vi "sv_Check for Even-Angle Signal.vi"(0 "data to process":waveform(dbl)[](array[waveform]), 11 "error in (no error)":errorcluster) -> (4 "data to process out":waveform(dbl)[](array[waveform]), 6 "even-angle signals":cluster{"r0":dbl, "dr":dbl, "Y":dbl[]}[](array[cluster]), 8 "even-angle channel info":T1[](array[typedef]) {"channel info"."pregain" format="%.2f"; "channel info"."weighting filter" items=["Linear", "A-weighting", "B-weighting", "C-weighting", "ITU-R 468-4", "Dolby", "CCITT", "C-message", "Wb", "Wc", "Wd", "We", "Wf", "Wh", "Wj", "Wk", "Wm", "AES17 20 kHz lowpass", "AES17 40 kHz lowpass", "AES17 20 kHz highpass", "AES17 40 kHz highpass"]; "channel info"."dB reference" format="%^.1e"; "channel info"."engineering units" items=["custom..."=0, "V"=1, "A"=21, "C"=30, "pC"=31, "s"=32, "-"=29, "Pa"=2, "N"=20, "g"=3, "m/s^2"=4, "m/s"=5, "m"=6, "mm/s"=12, "mm"=13, "micron/s"=14, "micron"=15, "in/s^2"=7, "in/s"=8, "in"=9, "mil/s"=10, "mil"=11, "rad/s^2"=16, "rad/s"=17, "rad"=18, "deg/s^2"=26, "deg/s"=27, "deg"=28, "RPM"=22, "cycle/s^2"=23, "Hz"=24, "cycle"=25, "strain"=19]; "channel info"."sensor sensitivity" format="%#_5f"}, 10 "even-angle position info":T5, 14 "found":bool, 15 "error out":errorcluster)   [LabVIEW 2017, in "SoundVib_ContSweptSine.lvlib"]
uses:
  <vilib>/addons/Sound and Vibration/svt_Continuous Swept Sine/SoundVib_ContSweptSine.lvlib
  <vilib>/addons/_NISVFA/_Shared subVIs/Controls/svc_Resampled Channel Info.ctl
  <vilib>/addons/_NISVFA/_Shared subVIs/Controls/svc_Channel Info.ctl
  <vilib>/addons/_NISVFA/_Shared subVIs/Controls/svc_Engineering Units Text Ring.ctl
  <vilib>/addons/_NISVFA/_Shared subVIs/Controls/svc_Weighting Filter Text Ring.ctl
  <vilib>/addons/Sound and Vibration/Order Analysis/Misc/OAT Position Info.ctl
  <vilib>/addons/Sound and Vibration/svt_Continuous Swept Sine/subVIs/sv_Continuous Swept-Sine Tags.ctl
  <vilib>/addons/Sound and Vibration/svt_Continuous Swept Sine/subVIs/sv_Continuous Swept-Sine Errors.ctl
panel:
  in  "even-angle position info":T5
  in  "even-angle channel info":T1[](array[typedef]) {"channel info"."pregain" format="%.2f"; "channel info"."weighting filter" items=["Linear", "A-weighting", "B-weighting", "C-weighting", "ITU-R 468-4", "Dolby", "CCITT", "C-message", "Wb", "Wc", "Wd", "We", "Wf", "Wh", "Wj", "Wk", "Wm", "AES17 20 kHz lowpass", "AES17 40 kHz lowpass", "AES17 20 kHz highpass", "AES17 40 kHz highpass"]; "channel info"."dB reference" format="%^.1e"; "channel info"."engineering units" items=["custom..."=0, "V"=1, "A"=21, "C"=30, "pC"=31, "s"=32, "-"=29, "Pa"=2, "N"=20, "g"=3, "m/s^2"=4, "m/s"=5, "m"=6, "mm/s"=12, "mm"=13, "micron/s"=14, "micron"=15, "in/s^2"=7, "in/s"=8, "in"=9, "mil/s"=10, "mil"=11, "rad/s^2"=16, "rad/s"=17, "rad"=18, "deg/s^2"=26, "deg/s"=27, "deg"=28, "RPM"=22, "cycle/s^2"=23, "Hz"=24, "cycle"=25, "strain"=19]; "channel info"."sensor sensitivity" format="%#_5f"}
  in  "even-angle signals":cluster{"r0":dbl, "dr":dbl, "Y":dbl[]}[](array[cluster]) {"r0" format="%.2p"; "dr" format="%.2p"; "Y" format="%.2f"}
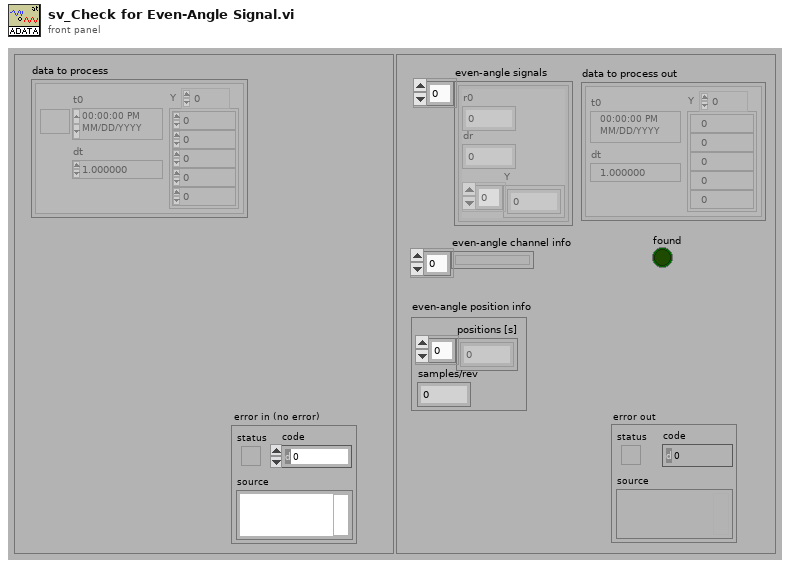
[diagram p1: front panel]
types:
  T1 = typedef "svc_Resampled Channel Info.ctl" = cluster{"channel name":string, "description":string, " channel info":T2}
  T2 = typedef "svc_Channel Info.ctl" = cluster{"sensor sensitivity":dbl, "engineering units":T3, "dB reference":dbl, "custom label":string, "weighting filter":T4, "pregain":dbl}
  T3 = typedef "svc_Engineering Units Text Ring.ctl" = u16
  T4 = typedef "svc_Weighting Filter Text Ring.ctl" = u16
  T5 = typedef "OAT Position Info.ctl" = cluster{"positions [s]":dbl[], "samples/rev":dbl}
  T6 = typedef "SoundVib_ContSweptSine.lvlib/sv_Continuous Swept-Sine Tags.ctl" = enum16{"samplesPerRevolution", "t2aPositions", "a2tPositions", "evenAngleSignal", "evenAnglePositionInfo", "evenAngleChannelInfo"}
  T7 = typedef "SoundVib_ContSweptSine.lvlib/sv_Continuous Swept-Sine Errors.ctl" = enum16{"Invalid AI sampling rate", "Item not found", "Invalid initial phase"}
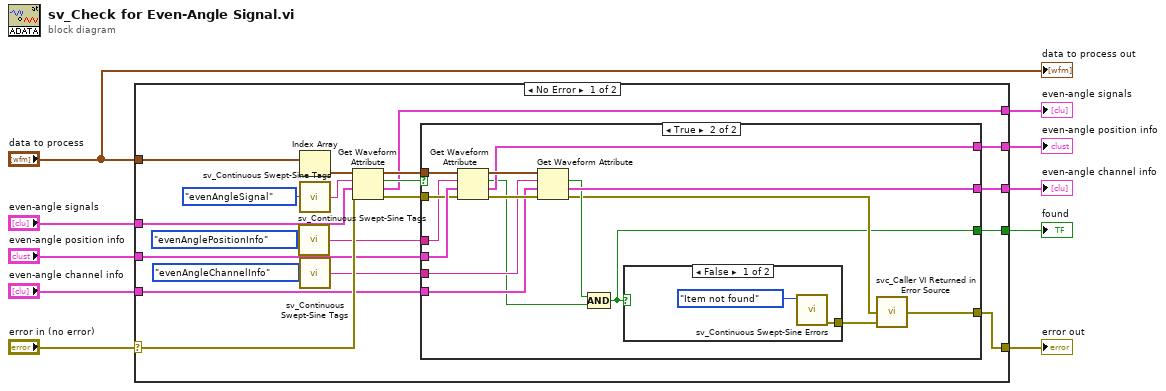
[diagram p0: block diagram]
diagram:
  n1 = case shown="No Error" "error in (no error)" {
    selector: "error in (no error)" -> [w25 w55]
    tunnel: [w12 w55] -> w9
    tunnel: "even-angle signals" -> [w28 w54]
    tunnel: "even-angle position info" -> [w21 w53]
    tunnel: "even-angle channel info" -> [w15 w52]
    tunnel: "data to process" -> [w30 _]
    tunnel: [w22 w54] -> w4
    tunnel: [w14 w53] -> w3
    tunnel: [w13 w52] -> w2
    tunnel: [w11 _] -> w1
    frame No Error {
      n2 = call <vilib>:"sv_Continuous Swept-Sine Tags.vi"("chirp sweep tag selector"=sv_Continuous_Swept-Sine_Tags."evenAnglePositionInfo" ("chirp sweep error selector")) -> ("Tag"=w18:string)
      n3 = Index Array(array=w30) -> (element=w29:waveform(dbl))  [unwired: 1 in]
      n4 = call <vilib>:"sv_Continuous Swept-Sine Tags.vi"("chirp sweep tag selector"=sv_Continuous_Swept-Sine_Tags."evenAngleSignal" ("chirp sweep error selector")) -> ("Tag"=w26:string)
      n5 = call <vilib>:"sv_Continuous Swept-Sine Tags.vi"("chirp sweep tag selector"=sv_Continuous_Swept-Sine_Tags."evenAngleChannelInfo" ("chirp sweep error selector")) -> ("Tag"=w16:string)
      n6 = Get Waveform Attribute(4:w25, 5:w28, 6:w26, 7:w29) -> (0:w20:errorcluster, 1:w22:cluster{"r0":dbl, "dr":dbl, "Y":dbl[]}[], 2:w24:bool, 3:w23:waveform(dbl))
      n7 = case shown="True" w24 {
        tunnel: w23 -> [_ w49]
        tunnel: w21 -> [w33 w48]
        tunnel: w20 -> [w31 w47]
        tunnel: w18 -> [_ w46]
        tunnel: w16 -> [_ w43]
        tunnel: w15 -> [w32 w42]
        tunnel: [w33 w41] -> w14
        tunnel: [w32 w40] -> w13
        tunnel: [w31 w35] -> w12
        tunnel: [_ w34] -> w11
        frame False {
        }
        frame True {
          n8 = Get Waveform Attribute(4:w47, 5:w48, 6:w46, 7:w49) -> (0:w44:errorcluster, 1:w41:T5, 2:w38:bool, 3:w45:waveform(dbl))
          n9 = Get Waveform Attribute(4:w44, 5:w42, 6:w43, 7:w45) -> (0:w37:errorcluster, 1:w40:T1[], 2:w39:bool)  [unwired: 1 out]
          n10 = Compound Arithmetic op=AND(w39, w38) -> (w34:bool)
          n11 = case shown="False" w34 {
            tunnel: [w50 _] -> w36
            frame False {
              n12 = call <vilib>:"sv_Continuous Swept-Sine Errors.vi"("continuous swept-sine error"=sv_Continuous_Swept-Sine_Errors."Item not found" ("chirp sweep error selector")) -> ("error out"=w50:errorcluster)  [unwired: 10 in]
            }
            frame True {
            }
          }
          n13 = call <vilib>:"svc_Caller VI Returned in Error Source.vi"("warning input to caller"=w36, "error in (no error)"=w37) -> ("error out"=w35:errorcluster)  [unwired: 3 in]
        }
      }
    }
    frame Error {
    }
  }
  "error out" <- w9
  "even-angle signals" <- w4
  "even-angle position info" <- w3
  "even-angle channel info" <- w2
  "found" <- w1
  "data to process out" <- "data to process"
